vi "De-Initialize.vi"(8 "error in (no error)":errorcluster, 11 "Micron sm Digitizer in":refnum<class "Micron sm Digitizer.lvclass">) -> (0 "error out":errorcluster, 3 "Micron sm Digitizer out":refnum<class "Micron sm Digitizer.lvclass">)   [LabVIEW 2024, in "Micron sm Digitizer.lvclass"]
uses:
  Micron sm Digitizer.lvclass
  Micron sm Digitizer.lvclass/Micron sm Digitizer.ctl
  Micron Optics sm130/Micron Optics sm130.lvlib
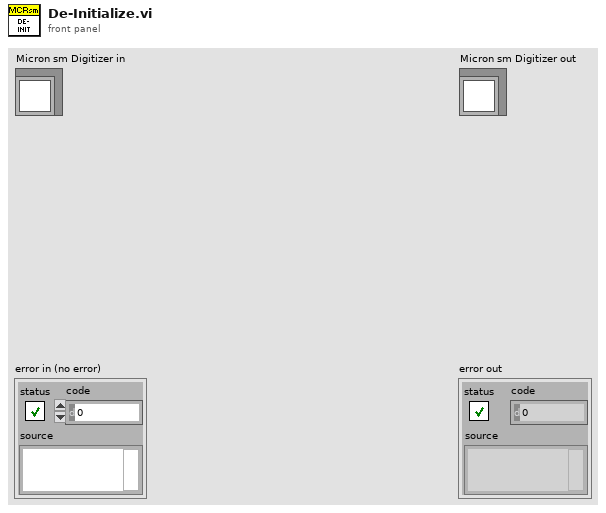
[diagram p1: front panel]
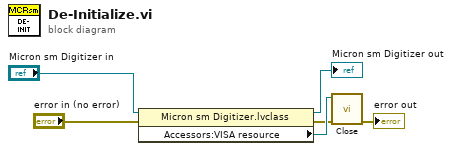
[diagram p0: block diagram]
diagram:
  n1 = property class="Micron sm Digitizer.lvclass"(reference="Micron sm Digitizer in", error in="error in (no error)") -> (reference out=→"Micron sm Digitizer out":refnum<class "Micron sm Digitizer.lvclass">, error out=w3:errorcluster, "Accessors:VISA resource"=w4:refnum<visa-resource-name>)
  n2 = call "Close.vi"("error in (no error)"=w3, "VISA resource name"=w4) -> ("error out"=→"error out":errorcluster)  [unwired: 9 in]
